vi "Configure Measurement.vi"(6 "Manual Range (1.00)":dbl=1.0 format="%_3f", 7 "Absolute Resolution (0: 5.5 Rate:Slow)":u16(ring) items=["5.5 Rate:Slow", "4.5 Rate:Middle", "4.5 Rate:Fast", "3.5 Rate", "6.5 Rate"], 8 "error in (no error)":errorcluster, 9 "Auto Range (T:Enable)":bool=TRUE, 10 "Function (0: DC Volts)":u16(ring) items=["DC Volts", "AC Volts", "DC Current", "AC Current", "2-Wire Resistance", "4-Wire Resistance", "Frequency", "Period", "Continuity", "Diode", "Capacitance", "Ratio"], 11 "VISA resource name":refnum<visa-resource-name>) -> (0 "error out":errorcluster, 3 "VISA resource name out":refnum<visa-resource-name>)   [LabVIEW 2020, in "Library Instrument & Equipement.lvlib" / "Library Multimeter.lvlib" / "RIGOL DM3058.lvlib"]
doc: "Configures the measurement type, resolution, and range on the instrument."
uses:
  RIGOL DM3058.lvlib
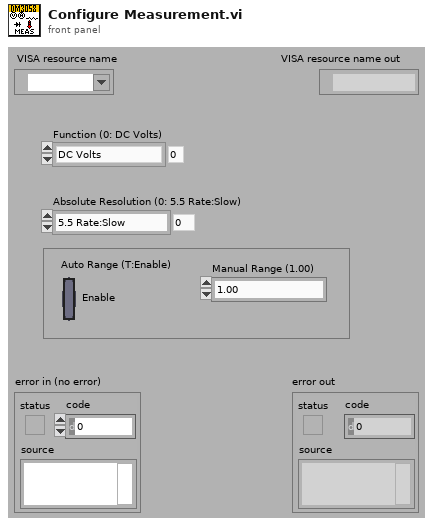
[diagram p1: front panel]
types:
  T1 = cluster{"DM Series Mode":u16, "Measurement Function":u16}
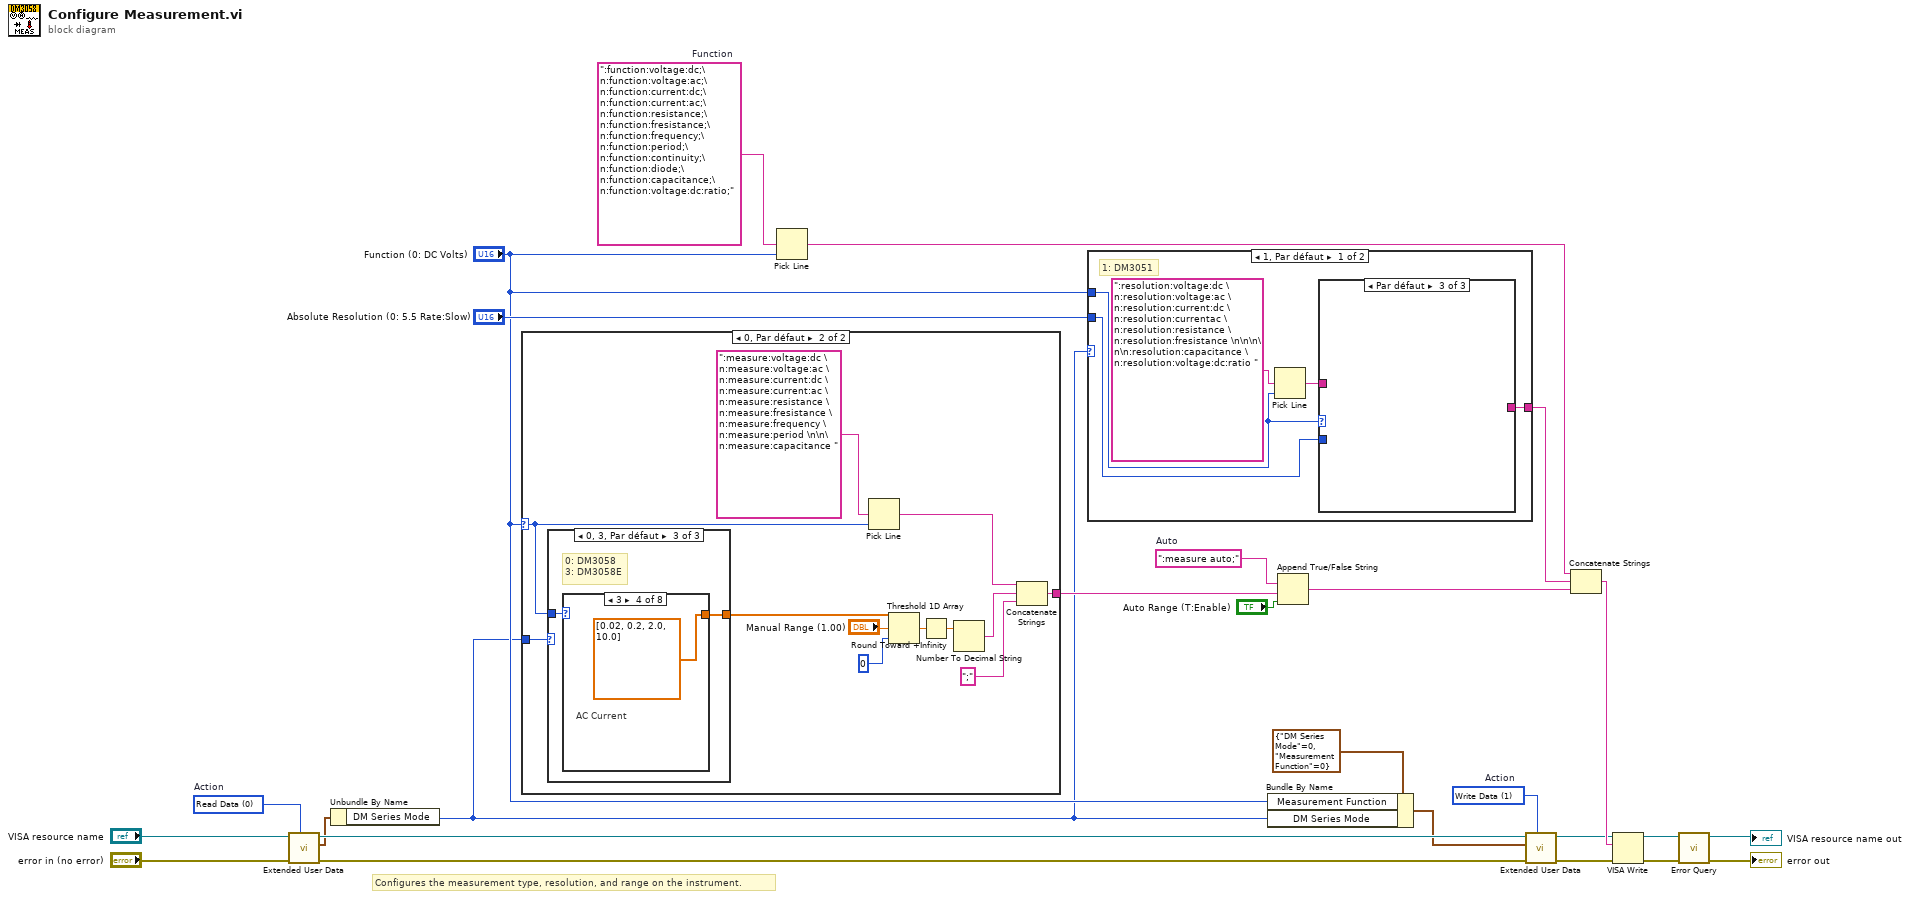
[diagram p0: block diagram]
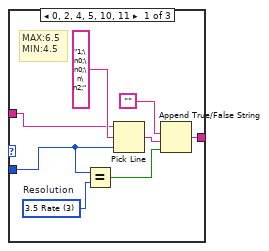
[diagram p2: hidden frame]
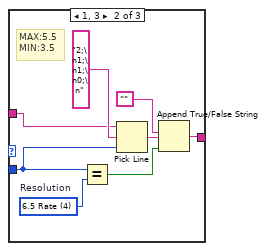
[diagram p3: hidden frame]
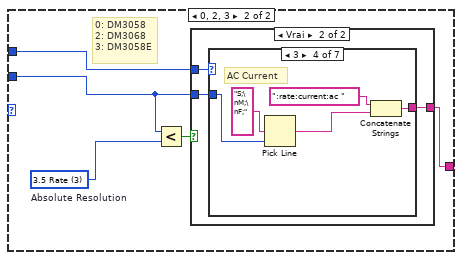
[diagram p4: hidden frame]
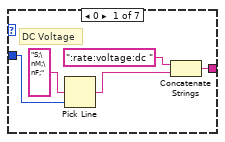
[diagram p6: hidden frame]
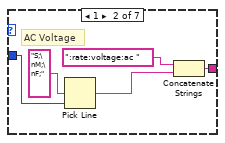
[diagram p7: hidden frame]
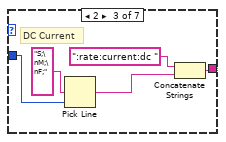
[diagram p8: hidden frame]
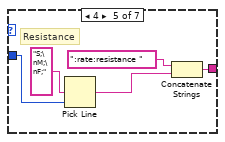
[diagram p9: hidden frame]
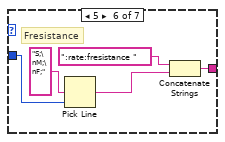
[diagram p10: hidden frame]
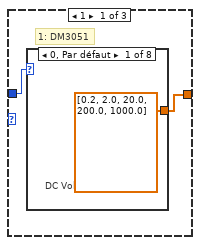
[diagram p13: hidden frame]
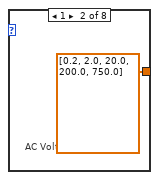
[diagram p14: hidden frame]
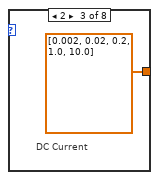
[diagram p15: hidden frame]
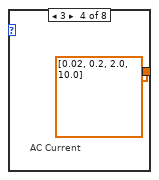
[diagram p16: hidden frame]
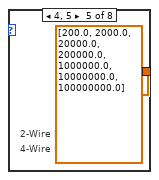
[diagram p17: hidden frame]
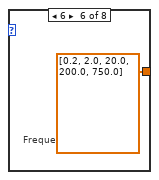
[diagram p18: hidden frame]
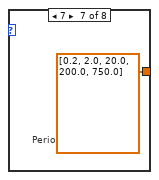
[diagram p19: hidden frame]
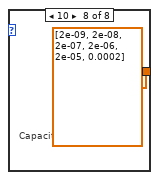
[diagram p20: hidden frame]
diagram:
  w10 = 1 items=["Read Data", "Write Data", "Clear Data", "Clear ALL Data"]  # Action
  w17 = 0 items=["Read Data", "Write Data", "Clear Data", "Clear ALL Data"]  # Action
  w23 = ":measure auto;"  # Auto
  w26 = ":function:voltage:dc;\n:function:voltage:ac;\n:function:current:dc;\n:function:current:ac;\n:function:resistance;\n:function:fresistance;\n:function:frequency;\n:function:period;\n:function:continuity;\n:function:diode;\n:function:capacitance;\n:function:voltage:dc:ratio;"  # Function
  # "Configures the measurement type, resolution, and range on the instrument."
  n1 = call "Extended User Data.vi"("Action (1: Write Data)"=w17, "Error In (no error)"="error in (no error)", "VISA resource name in"="VISA resource name") -> ("Error Out"=w12:errorcluster, "User Data Out"=w3:T1, "VISA resource name out"=w14:refnum<visa-resource-name>)  [unwired: 1 in, 5 out]
  n2 = Unbundle By Name(w3) -> ("DM Series Mode"=w4:u16)
  n3 = case shown="0, Par défaut" "Function (0: DC Volts)" {
    selector: "Function (0: DC Volts)" -> [_ w31]
    tunnel: [_ w28] -> w22
    tunnel: w4 -> [_ w27]
    frame 8, 9, 11 {
      # "Continuity, Diode and Ratio functions don't have manual range setting."
    }
    frame 0, Default {
      n4 = case shown="0, 3, Par défaut" w27 {
        tunnel: [w40 w49 w60] -> w35
        tunnel: w31 -> [w39 w50 w59]
        frame 1 {
          # "1: DM3051"
          n5 = case shown="0, Par défaut" w39 {
            tunnel: [dbl[] [0.2, 2.0, 20.0, 200.0, 1000.0] ("Array Constant") dbl[] [0.2, 2.0, 20.0, 200.0, 750.0] ("Array Constant") dbl[] [0.002, 0.02, 0.2, 1.0, 10.0] ("Array Constant") dbl[] [0.02, 0.2, 2.0, 10.0] ("Array Constant") dbl[] [200.0, 2000.0, 20000.0, 200000.0, 1000000.0, 10000000.0, 100000000.0] ("Array Constant") dbl[] [0.2, 2.0, 20.0, 200.0, 750.0] ("Array Constant") dbl[] [0.2, 2.0, 20.0, 200.0, 750.0] ("Array Constant") dbl[] [2e-09, 2e-08, 2e-07, 2e-06, 2e-05, 0.0002] ("Array Constant")] -> w40
            frame 0, Default {
              # "DC Voltage"
            }
            frame 1 {
              # "AC Voltage"
            }
            frame 2 {
              # "DC Current"
            }
            frame 3 {
              # "AC Current"
            }
            frame 4, 5 {
              # "4-Wire Resis."
              # "2-Wire Resis."
            }
            frame 6 {
              # "Frequency"
            }
            frame 7 {
              # "Period"
            }
            frame 10 {
              # "Capacitance"
            }
          }
        }
        frame 2 {
          # "2: DM3068"
          n6 = case shown="0, Par défaut" w50 {
            tunnel: [dbl[] [0.2, 2.0, 20.0, 200.0, 1000.0] ("Array Constant") dbl[] [0.2, 2.0, 20.0, 200.0, 750.0] ("Array Constant") dbl[] [0.0002, 0.002, 0.02, 0.2, 2.0, 10.0] ("Array Constant") dbl[] [0.0002, 0.002, 0.02, 0.2, 2.0, 20.0] ("Array Constant") dbl[] [200.0, 2000.0, 20000.0, 200000.0, 1000000.0, 10000000.0, 100000000.0] ("Array Constant") dbl[] [0.2, 2.0, 20.0, 200.0, 750.0] ("Array Constant") dbl[] [0.2, 2.0, 20.0, 200.0, 750.0] ("Array Constant") dbl[] [2e-09, 2e-08, 2e-07, 2e-06, 2e-05, 0.0002, 0.002, 0.02, 0.1] ("Array Constant")] -> w49
            frame 0, Default {
              # "DC Voltage"
            }
            frame 1 {
              # "AC Voltage"
            }
            frame 2 {
              # "DC Current"
            }
            frame 3 {
              # "AC Current"
            }
            frame 4, 5 {
              # "4-Wire Resis."
              # "2-Wire Resis."
            }
            frame 6 {
              # "Frequency"
            }
            frame 7 {
              # "Period"
            }
            frame 10 {
              # "Capacitance"
            }
          }
        }
        frame 0, 3, Default {
          # "0: DM3058\n3: DM3058E"
          n7 = case shown="3" w59 {
            tunnel: [dbl[] [0.2, 2.0, 20.0, 200.0, 1000.0] ("Array Constant") dbl[] [0.2, 2.0, 20.0, 200.0, 750.0] ("Array Constant") dbl[] [0.0002, 0.002, 0.02, 0.2, 2.0, 10.0] ("Array Constant") dbl[] [0.02, 0.2, 2.0, 10.0] ("Array Constant") dbl[] [200.0, 2000.0, 20000.0, 200000.0, 2000000.0, 10000000.0, 100000000.0] ("Array Constant") dbl[] [0.2, 2.0, 20.0, 200.0, 750.0] ("Array Constant") dbl[] [0.2, 2.0, 20.0, 200.0, 750.0] ("Array Constant") dbl[] [2e-09, 2e-08, 2e-07, 2e-06, 0.0002, 0.01] ("Array Constant")] -> w60
            frame 0, Default {
              # "DC Voltage"
            }
            frame 1 {
              # "AC Voltage"
            }
            frame 2 {
              # "DC Current"
            }
            frame 3 {
              # "AC Current"
            }
            frame 4, 5 {
              # "4-Wire Resis."
              # "2-Wire Resis."
            }
            frame 6 {
              # "Frequency"
            }
            frame 7 {
              # "Period"
            }
            frame 10 {
              # "Capacitance"
            }
          }
        }
      }
      n8 = Pick Line(multi-line string=":measure:voltage:dc \n:measure:voltage:ac \n:measure:current:dc \n:measure:current:ac \n:measure:resistance \n:measure:fresistance \n:measure:frequency \n:measure:period \n\n\n:measure:capacitance ", line index=w31) -> (output string=w30:string)  [unwired: 1 out]
      n9 = Threshold 1D Array(1:0 ("start index (0)"), 2:"Manual Range (1.00)", 3:w35) -> (0:w36:dbl)
      n10 = Round Toward +Infinity ("Round To +Infinity")(x=w36) -> (ceil(x): smallest int >= x=w34:dbl)
      n11 = Number To Decimal String(number=w34) -> (decimal integer string=w33:string)  [unwired: 1 out]
      n12 = Concatenate Strings(w30, w33, ";" ("字符串")) -> (w28:string)
    }
  }
  n13 = Pick Line(multi-line string=w26, line index="Function (0: DC Volts)") -> (output string=w15:string)  [unwired: 1 out]
  n14 = case shown="1, Par défaut" w4 {
    tunnel: "Absolute Resolution (0: 5.5 Rate:Slow)" -> [w72 w91]
    tunnel: "Function (0: DC Volts)" -> [w73 w94]
    tunnel: [w69 w93] -> w16
    frame 1, Default {
      # "1: DM3051"
      n15 = Pick Line(multi-line string=":resolution:voltage:dc \n:resolution:voltage:ac \n:resolution:current:dc \n:resolution:currentac \n:resolution:resistance \n:resolution:fresistance \n\n\n\n\n:resolution:capacitance \n:resolution:voltage:dc:ratio " ("string (\"\")"), line index=w73) -> (output string=w70:string)  [unwired: 1 out]
      n16 = case shown="Par défaut" w73 {
        tunnel: w72 -> [w79 w83 _]
        tunnel: w70 -> [w80 w88 _]
        tunnel: [w77 w85 _] -> w69
        frame 0, 2, 4, 5, 10, 11 {
          w78 = u16 3 items=["5.5 Rate:Slow", "4.5 Rate:Middle", "4.5 Rate:Fast", "3.5 Rate", "6.5 Rate"]  # Resolution
          # "MAX:6.5\nMIN:4.5"
          n17 = Equal?(x=w79, y=w78) -> (x = y?=w76:bool)
          n18 = Pick Line(string ("")=w80, multi-line string="1;\n0;\n0;\n\n2;", line index=w79) -> (output string=w75:string)
          n19 = Append True/False String(1:w76, 2:w75, 3:"") -> (0:w77:string)  [unwired: 1 out]
        }
        frame 1, 3 {
          w87 = u16 4 items=["5.5 Rate:Slow", "4.5 Rate:Middle", "4.5 Rate:Fast", "3.5 Rate", "6.5 Rate"]  # Resolution
          # "MAX:5.5\nMIN:3.5"
          n20 = Equal?(x=w83, y=w87) -> (x = y?=w84:bool)
          n21 = Pick Line(string ("")=w88, multi-line string="2;\n1;\n1;\n0;\n", line index=w83) -> (output string=w86:string)
          n22 = Append True/False String(1:w84, 2:w86, 3:"") -> (0:w85:string)  [unwired: 1 out]
        }
        frame Default {
        }
      }
    }
    frame 0, 2, 3 {
      w92 = u16 3 items=["5.5 Rate:Slow", "4.5 Rate:Middle", "4.5 Rate:Fast", "3.5 Rate", "6.5 Rate"]  # Absolute Resolution
      # "0: DM3058\n2: DM3068\n3: DM3058E"
      n23 = Less?(x=w91, y=w92) -> (x < y?=w90:bool)
      n24 = case shown="Vrai" w90 {
        tunnel: w94 -> [_ w97]
        tunnel: [_ w96] -> w93
        tunnel: w91 -> [_ w95]
        frame False {
          # "The DM3058 and DM3068 don't \nsupport 3.5 Rate and 6.5 Rate \noptions."
        }
        frame True {
          n25 = case shown="3" w97 {
            tunnel: w95 -> [w101 w106 w111 w116 w121 w126 _]
            tunnel: [w98 w103 w108 w113 w118 w123 _] -> w96
            frame 0 {
              # "DC Voltage"
              n26 = Pick Line(multi-line string="S;\nM;\nF;", line index=w101) -> (output string=w100:string)  [unwired: 1 out]
              n27 = Concatenate Strings(":rate:voltage:dc ", w100) -> (w98:string)
            }
            frame 1 {
              # "AC Voltage"
              n28 = Pick Line(multi-line string="S;\nM;\nF;", line index=w106) -> (output string=w105:string)  [unwired: 1 out]
              n29 = Concatenate Strings(":rate:voltage:ac ", w105) -> (w103:string)
            }
            frame 2 {
              # "DC Current"
              n30 = Pick Line(multi-line string="S;\nM;\nF;", line index=w111) -> (output string=w110:string)  [unwired: 1 out]
              n31 = Concatenate Strings(":rate:current:dc ", w110) -> (w108:string)
            }
            frame 3 {
              # "AC Current"
              n32 = Pick Line(multi-line string="S;\nM;\nF;", line index=w116) -> (output string=w115:string)  [unwired: 1 out]
              n33 = Concatenate Strings(":rate:current:ac ", w115) -> (w113:string)
            }
            frame 4 {
              # "Resistance"
              n34 = Pick Line(multi-line string="S;\nM;\nF;", line index=w121) -> (output string=w120:string)  [unwired: 1 out]
              n35 = Concatenate Strings(":rate:resistance ", w120) -> (w118:string)
            }
            frame 5 {
              # "Fresistance"
              n36 = Pick Line(multi-line string="S;\nM;\nF;", line index=w126) -> (output string=w125:string)  [unwired: 1 out]
              n37 = Concatenate Strings(":rate:fresistance ", w125) -> (w123:string)
            }
            frame 6, Default {
              # "DM3058, DM3068:\nfrequency period continuity diode \ncapacitance functions can't set \nrate"
            }
          }
        }
      }
    }
  }
  n38 = Bundle By Name(cluster=T1 {"DM Series Mode"=0, "Measurement Function"=0} ("User Data Out"), "Measurement Function"="Function (0: DC Volts)", "DM Series Mode"=w4) -> (w1:T1)
  n39 = Append True/False String(1:"Auto Range (T:Enable)", 2:w22, 3:w23) -> (0:w21:string)  [unwired: 1 out]
  n40 = call "Extended User Data.vi"("Action (1: Write Data)"=w10, "Error In (no error)"=w12, "User Data In"=w1, "VISA resource name in"=w14) -> ("Error Out"=w11:errorcluster, "VISA resource name out"=w13:refnum<visa-resource-name>)  [unwired: 6 out]
  n41 = Concatenate Strings(w15, w16, w21) -> (w20:string)
  n42 = VISA Write(VISA resource name=w13, write buffer=w20, error in (no error)=w11) -> (VISA resource name out=w8:refnum<visa-resource-name>, error out=w7:errorcluster)  [unwired: 1 out]
  n43 = call "Error Query.vi"("error in (no error)"=w7, "VISA resource name"=w8) -> ("error out"=→"error out":errorcluster, "VISA resource name out"=→"VISA resource name out":refnum<visa-resource-name>)  [unwired: 8 out]
